vi "Camera Calibration to String.vi"(8 "error in (no error)":errorcluster, 10 "rectangle":T1 {"Rotation" format="%.2f"; "Left" scale=0.0..1024.0; "Right" scale=0.0..1024.0}, 11 "mm/pixel":dbl) -> (0 "error out":errorcluster, 3 "cam cal string":string)   [LabVIEW 2020]
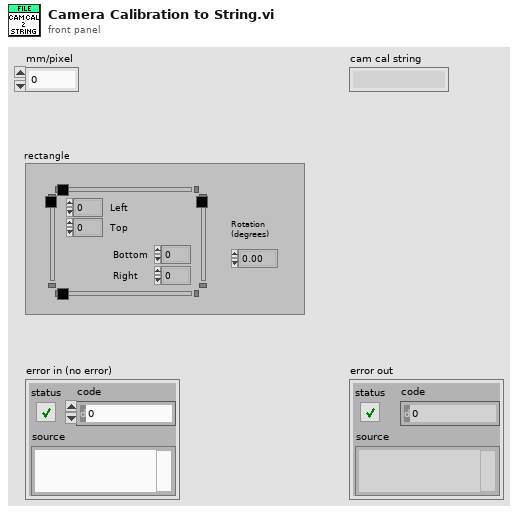
[diagram p1: front panel]
types:
  T1 = typedef "IMAQ Rectangle" = cluster{"Left":i32, "Top":i32, "Right":i32, "Bottom":i32, "Rotation":dbl}
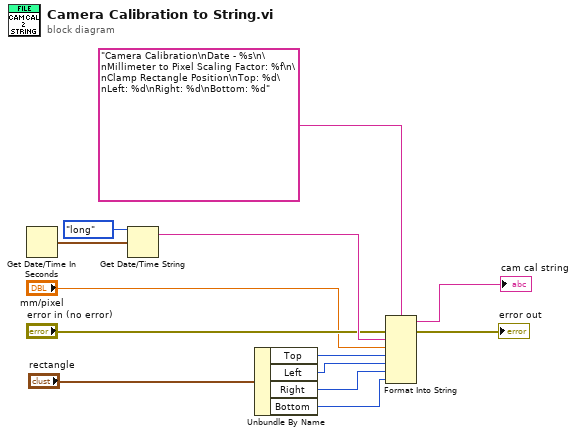
[diagram p0: block diagram]
diagram:
  n1 = Get Date/Time In Seconds() -> (seconds since 1Jan1904=w12:timestamp)
  n2 = Get Date/Time String(date format (0)=enum16{"short", "long", "abbreviated"}."long", seconds (now)=w12) -> (date string=w10:string)  [unwired: 1 in, 1 out]
  n3 = Unbundle By Name("rectangle") -> ("Top"=w5:i32, "Left"=w4:i32, "Right"=w3:i32, "Bottom"=w2:i32)
  n4 = Format Into String(format string="Camera Calibration\nDate - %s\n\nMillimeter to Pixel Scaling Factor: %f\n\nClamp Rectangle Position\nTop: %d\nLeft: %d\nRight: %d\nBottom: %d", error in="error in (no error)", w10, "mm/pixel", w5, w4, w3, w2) -> (resulting string=→"cam cal string":string, error out=→"error out":errorcluster)  [unwired: 1 in]
